vi "M Smart Grid.vi"(11 "EV3 in":T1) -> (3 "EV3 out":T1)   [LabVIEW 2016]
uses:
  <vilib>/NXT/Subs/LVHSConnector.ctl
  <vilib>/NXT/LegoClasses/BrickReference/BrickReference.lvclass
  <vilib>/NXT/Block Support/NXT_OutputPort.ctl
  <vilib>/NXT/NXTIO Xnodes/NXTIONodeSubVIs/NXTMoveMotors.vi
  <vilib>/NXT/Dual Mode Library/Waits/Wait_Num.vi
  <vilib>/NXT/NXTIO Xnodes/AddressXNode/NXTIOAddress.xnode
  <vilib>/NXT/NXTIO Xnodes/NXTIOXNode/NXTIO.xnode
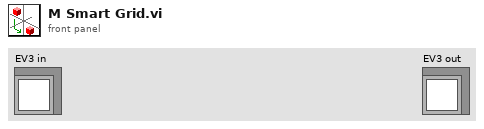
[diagram p1: front panel]
types:
  T1 = typedef "LVHSConnector.ctl" = refnum<class "BrickReference.lvclass">
  T2 = typedef "NXT_OutputPort.ctl" = u8
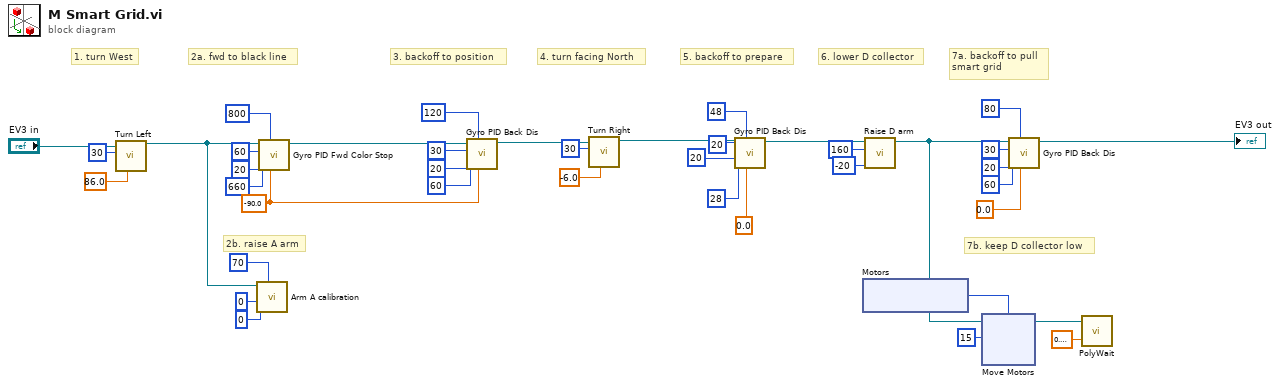
[diagram p0: block diagram]
diagram:
  w29 = sgl -90.0 ("Target angle")
  # "7b. keep D collector low"
  # "7a. backoff to pull\nsmart grid"
  # "6. lower D collector"
  # "5. backoff to prepare"
  # "4. turn facing North"
  # "3. backoff to position"
  # "2b. raise A arm"
  # "2a. fwd to black line"
  # "1. turn West"
  n1 = call "Turn Left.vi"("Turning angle"=sgl 86.0, "Motor B (right)"=i8 30, "EV3 in"="EV3 in") -> ("EV3 out"=w34:T1)  [unwired: 8 in]
  n2 = call "Arm A calibration.vi"("Cali. Power"=i8 70, "Down Power"=i8 0, "Rotation"=0, "NXT/EV3"=w34) -> ()  [unwired: 7 in, 1 out]
  n3 = call "Gyro PID Fwd Color Stop.vi"("Target angle"=w29, "Threshold to Color"=800, "Threshold to slow"=660, "Min. speed"=20, "Max. speed"=60, "EV3 in"=w34) -> ("EV3 out"=w7:T1)  [unwired: 5 in]
  n4 = call "Gyro PID Back Dis.vi"("Target angle"=w29, "Threshold to stop"=120, "Threshold to slow"=60, "Min. speed"=20, "Max. speed"=30, "EV3 in"=w7) -> ("EV3 out"=w28:T1)  [unwired: 5 in]
  n5 = call "Turn Right.vi"("Turning angle"=sgl -6.0, "Motor B (right)"=i8 30, "EV3 in"=w28) -> ("EV3 out"=w25:T1)  [unwired: 8 in]
  n6 = call "Gyro PID Back Dis.vi"("Target angle"=sgl 0.0, "Threshold to stop"=48, "Threshold to slow"=28, "Min. speed"=20, "Max. speed"=20, "EV3 in"=w25) -> ("EV3 out"=w19:T1)  [unwired: 5 in]
  n7 = xnode "Motors"() -> ("Motor"=w1:T2)
  n8 = call "Raise D arm.vi"("Power"=i8 -20, "Rotation"=160, "EV3 in"=w19) -> ("EV3 out"=w6:T1)  [unwired: 8 in]
  n9 = xnode "Move Motors"("Power/Speed 1"=i8 15, "Motors"=w1, "NXT/EV3"=w6) -> ("NXT/EV3"=w4:T1)
  n10 = call "Gyro PID Back Dis.vi"("Target angle"=sgl 0.0, "Threshold to stop"=80, "Threshold to slow"=60, "Min. speed"=20, "Max. speed"=30, "EV3 in"=w6) -> ("EV3 out"=→"EV3 out":T1)  [unwired: 5 in]
  n11 = call-poly <vilib>:"PolyWait.vi"("Time (1 sec)"=sgl 0.4, "NXT/EV3"=w4) -> ()  [unwired: 2 in, 1 out]
